vi "Global stack names.vi"() -> ()   [LabVIEW 2023]
uses:
  ctrl defs/ctrl stack - INTAKE SHOOTER.ctl
panel:
  in  "Tab Control":enum32{"INTAKE & SHOOTER"}(tab)
  in  "INTAKE SHOOTER stack":T1={"INTAKE STATE"="INTAKE/STATE", "RUN INTAKE?"="INTAKE/RUN?", "RUN REVERSE?"="INTAKE/REVERSE?", "NOTE LOADED?"="INTAKE/NOTE?", "SHOOTER STATE"="SHOOTER/STATE", "SHOOTER FIRE?"="SHOOTER/FIRE?", "SHOOT AMP?"="SHOOTER/AMP?", "EXTEND FLAP?"="SHOOTER/FLAP?", "LOOKING for NOTE"="INTAKE/SEARCHING", "OVERIDE NOTE CHECK"="SHOOTER/OVERIDE NOTE CHECK"}
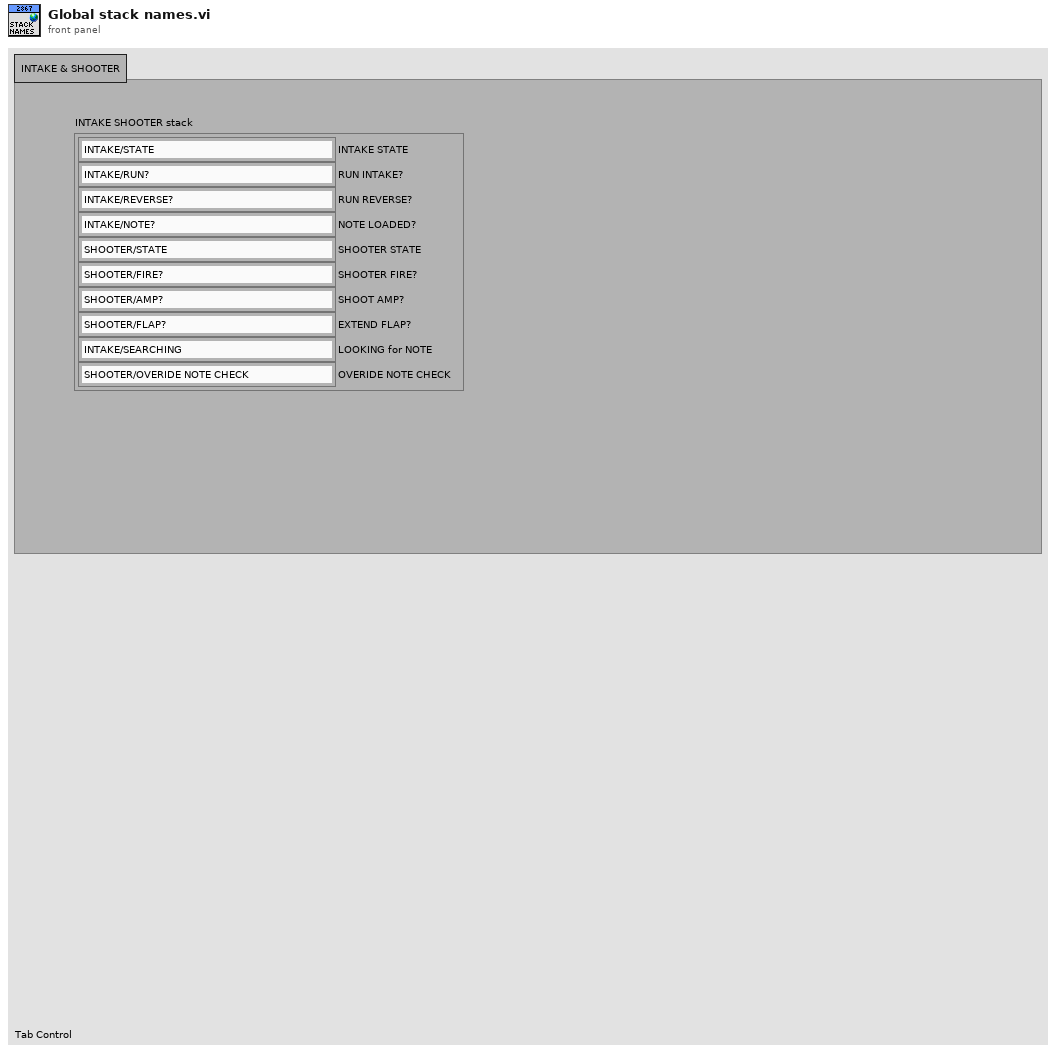
[diagram p1: front panel]
types:
  T1 = typedef "ctrl stack - INTAKE SHOOTER.ctl" = cluster{"INTAKE STATE":string, "RUN INTAKE?":string, "RUN REVERSE?":string, "NOTE LOADED?":string, "SHOOTER STATE":string, "SHOOTER FIRE?":string, "SHOOT AMP?":string, "EXTEND FLAP?":string, "LOOKING for NOTE":string, "OVERIDE NOTE CHECK":string}
diagram:
